vi "Heat2D_Cal Coeff.vi"(9 "a":dbl, 10 "k":dbl=1.0, 11 "Domain":T2) -> (1 "Matr_RHS":dbl[][](array[numeric]), 2 "Coefficients":T1, 3 "Domain Dup":T2, 4 "c != 0":bool)   [LabVIEW 2017, in "NI_PDE.lvlib"]
uses:
  <vilib>/gmath/NI_PDE.lvlib
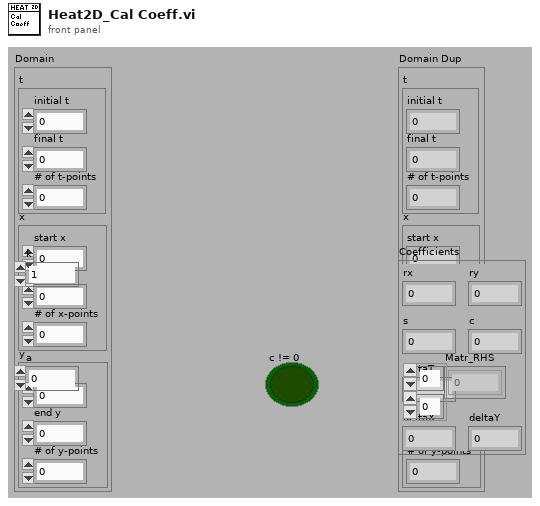
[diagram p1: front panel]
types:
  T1 = cluster{"rx":dbl, "ry":dbl, "s":dbl, "c":dbl, "deltaT":dbl, "deltaX":dbl, "deltaY":dbl}
  T2 = cluster{"t":cluster{"initial t":dbl, "final t":dbl, "# of t-points":i32}, "x":cluster{"start x":dbl, "end x":dbl, "# of x-points":i32}, "y":cluster{"start y":dbl, "end y":dbl, "# of y-points":i32}}
  T3 = cluster{"initial t":dbl, "final t":dbl, "# of t-points":i32}
  T4 = cluster{"start x":dbl, "end x":dbl, "# of x-points":i32}
  T5 = cluster{"start y":dbl, "end y":dbl, "# of y-points":i32}
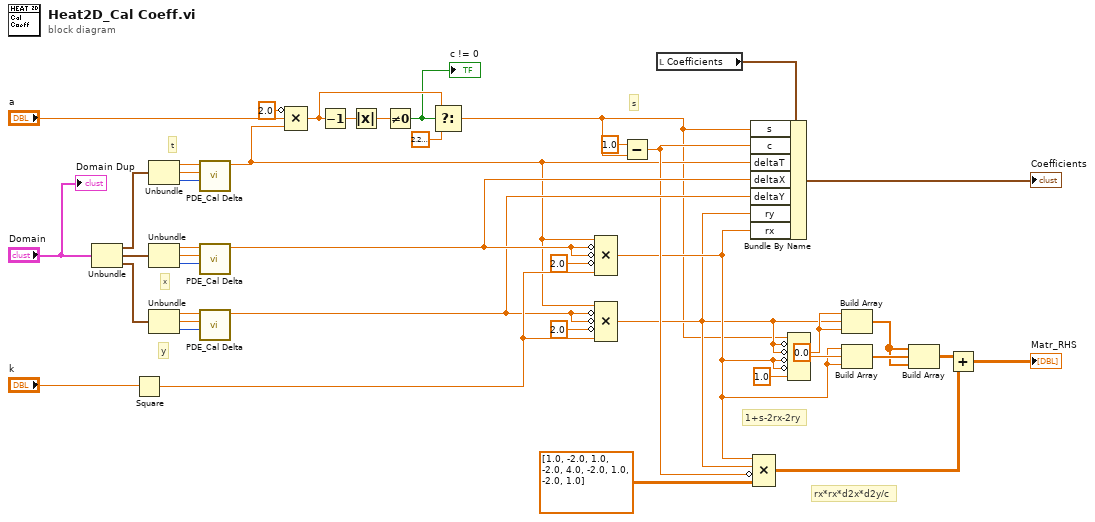
[diagram p0: block diagram]
diagram:
  w16 = 0.0 ("element")
  # "rx*rx*d2x*d2y/c"
  # "1+s-2rx-2ry"
  # "s"
  # "x"
  # "y"
  # "t"
  n1 = Unbundle("Domain") -> ("t"=w8:T3, "x"=w33:T4, "y"=w34:T5)
  n2 = Square(x="k") -> (x^2=w27:dbl)
  n3 = Unbundle(w8) -> ("initial t"=w41:dbl, "final t"=w42:dbl, "# of t-points"=w43:i32)
  n4 = Unbundle(w33) -> ("start x"=w38:dbl, "end x"=w39:dbl, "# of x-points"=w40:i32)
  n5 = Unbundle(w34) -> ("start y"=w35:dbl, "end y"=w36:dbl, "# of y-points"=w37:i32)
  n6 = call <vilib>:"PDE_Cal Delta.vi"("# of points"=w43, "end"=w42, "start"=w41) -> ("delta"=w6:dbl)  [unwired: 8 out]
  n7 = call <vilib>:"PDE_Cal Delta.vi"("# of points"=w40, "end"=w39, "start"=w38) -> ("delta"=w22:dbl)  [unwired: 8 out]
  n8 = call <vilib>:"PDE_Cal Delta.vi"("# of points"=w37, "end"=w36, "start"=w35) -> ("delta"=w21:dbl)  [unwired: 8 out]
  n9 = Compound Arithmetic op=MULTIPLY(invert 2.0 ("value"), "a", w6) -> (w3:dbl)
  n10 = Decrement(x=w3) -> (x-1=w30:dbl)
  n11 = Absolute Value(x=w30) -> (abs(x)=w5:dbl)
  n12 = Not Equal To 0?(x=w5) -> (x != 0?=w1:bool)
  "c != 0" <- w1
  n13 = Select(t=w3, s=w1, f=2.220446049250313e-16) -> (s? t:f=w2:dbl)
  n14 = Compound Arithmetic op=MULTIPLY(w6, invert w22, invert w22, invert 2.0 ("value"), w27) -> (w11:dbl)
  n15 = Compound Arithmetic op=MULTIPLY(w6, invert w21, invert w21, invert 2.0 ("value"), w27) -> (w10:dbl)
  n16 = Subtract(x=1.0, y=w2) -> (x-y=w12:dbl)
  n17 = local read "Coefficients"() -> (w24:T1)
  n18 = Bundle By Name(cluster=w24, "s"=w2, "c"=w12, "deltaT"=w6, "deltaX"=w22, "deltaY"=w21, "ry"=w10, "rx"=w11) -> (→"Coefficients":T1)
  n19 = Compound Arithmetic op=MULTIPLY(w11, w10, invert w12, dbl[][] [[1.0, -2.0, 1.0], [-2.0, 4.0, -2.0], [1.0, -2.0, 1.0]]) -> (w14:dbl[][])
  n20 = Compound Arithmetic op=ADD(w2, invert w10, invert w10, invert w11, invert w11, 1.0 ("value")) -> (w18:dbl)
  n21 = Build Array(w16, w10, w16) -> (w19:dbl[])
  n22 = Build Array(w11, w18, w11) -> (w20:dbl[])
  n23 = Build Array(w19, w20, w19) -> (w13:dbl[][])
  n24 = Add(x=w13, y=w14) -> (x+y=→"Matr_RHS":dbl[][])
  "Domain Dup" <- "Domain"
